vi "rs3 start w queue.vi"(0 "Sensor  in":u64, 1 "queue in":u64, 3 "error in (no error)":errorcluster) -> (7 "sensor out":u64, 8 "queue out":u64, 9 "error":u64, 10 "error out":errorcluster)   [LabVIEW 2019, in "libRealSense3.lvlib"]
doc: "STARTS the streaming of a specific sensor, based on the input QUEUE."
uses:
  libRealSense3.lvlib
  realsense2.dll
panel:
  # "RS Start Queue"
  # "(C) 2017 Intel Corp.,  AGJ"
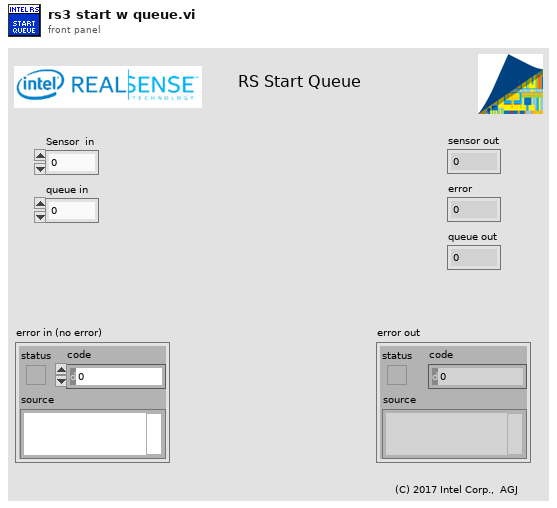
[diagram p1: front panel]
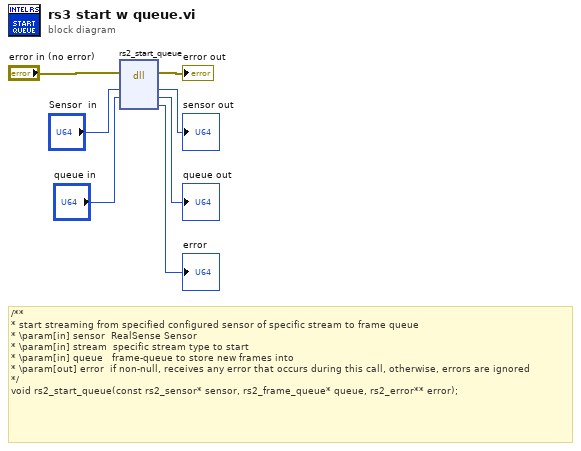
[diagram p0: block diagram]
diagram:
  # "/**\n* start streaming from specified configured sensor of specific stream to frame queue\n* \\param[in] sensor  RealSense Sensor\n* \\param[in] stream  specific stream type to start\n* \\param[in] queue   frame-queue to store new frames into\n* \\param[out] error  if non-null, receives any error that occurs during this call, otherwise, errors are ignored\n*/\nvoid rs2_start_queue(const rs2_sensor* sensor, rs2_frame_queue* queue, rs2_error** error);"
  n1 = dll-call lib="C:/Users/morte/Documents/gitmoro/treadmill/RealSense for Labview ver. 2.33/realsense2.dll" fn="rs2_start_queue"(error in="error in (no error)", "sensor in"="Sensor  in", "queue"="queue in") -> (error out=→"error out":errorcluster, "sensor in"=→"sensor out":u64, "queue"=→"queue out":u64, "error"=→"error":u64)  [unwired: 4 in, 1 out]
